vi "Write Calculated Delay.vi"(8 "error in (no error)":errorcluster, 10 "Calculated Delay":dbl[](array[numeric]), 11 "Readout Charact in":refnum<class "Readout Charact.lvclass">) -> (0 "error out":errorcluster, 3 "Readout Charact out":refnum<class "Readout Charact.lvclass">)   [LabVIEW 2018, in "Readout Charact.lvclass"]
uses:
  Readout Charact.lvclass
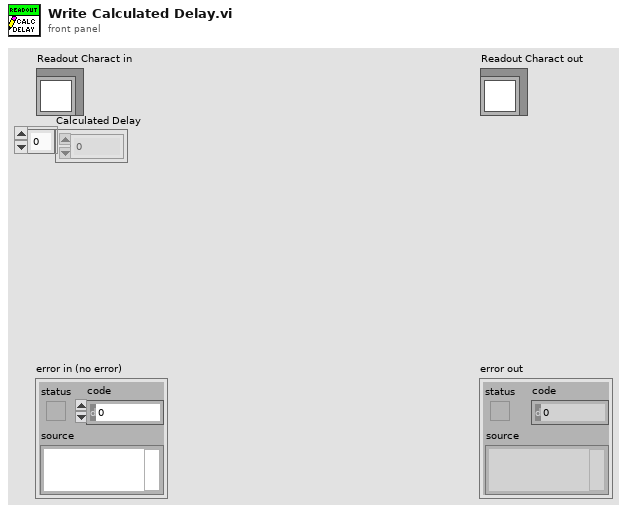
[diagram p1: front panel]
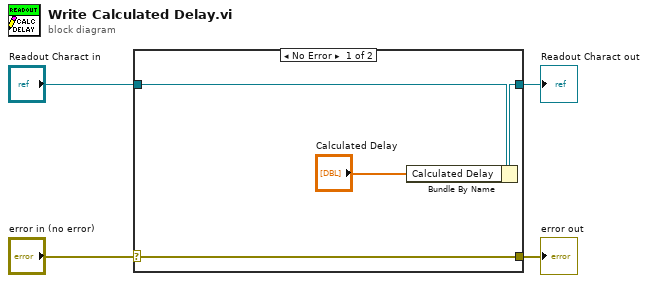
[diagram p0: block diagram]
diagram:
  n1 = case shown="No Error" "error in (no error)" {
    selector: "error in (no error)" -> [w8 w9]
    tunnel: [w8 w9] -> w3
    tunnel: [w6 w10] -> w1
    tunnel: "Readout Charact in" -> [w7 w10]
    frame No Error {
      n2 = Bundle By Name(cluster=w7, "Calculated Delay"="Calculated Delay") -> (w6:refnum<class "Readout Charact.lvclass">)
    }
    frame Error {
    }
  }
  "error out" <- w3
  "Readout Charact out" <- w1
